vi "configure.vi"(8 "error in (no error)":errorcluster, 11 "ImagingModeDL100901FlexTrajectory in":refnum<class "ImagingModeDL100901FlexTrajectory.lvclass">) -> (0 "error out":errorcluster, 3 "ImagingModeDL100901FlexTrajectory out":refnum<class "ImagingModeDL100901FlexTrajectory.lvclass">)   [LabVIEW 2010, in "ImagingModeDL100901FlexTrajectory.lvclass"]
doc: "The dynamic dispatch version of this VI loads and displays the configuration file associated with the plug-in object. The user modify and save the configuration data."
uses:
  ImagingModeDL100901FlexTrajectory.lvclass
  ImagingModeDL090923Scaffold/ImagingModeDL090923Scaffold/configuration_visibility_cluster.ctl
  ImagingModeDL090923Scaffold/ImagingModeDL090923Scaffold/component_configuration_visibility_cluster.ctl
  ImagingModeDL090923Scaffold/ImagingModeDL090923Scaffold/ImagingModeDL090923Scaffold.lvclass
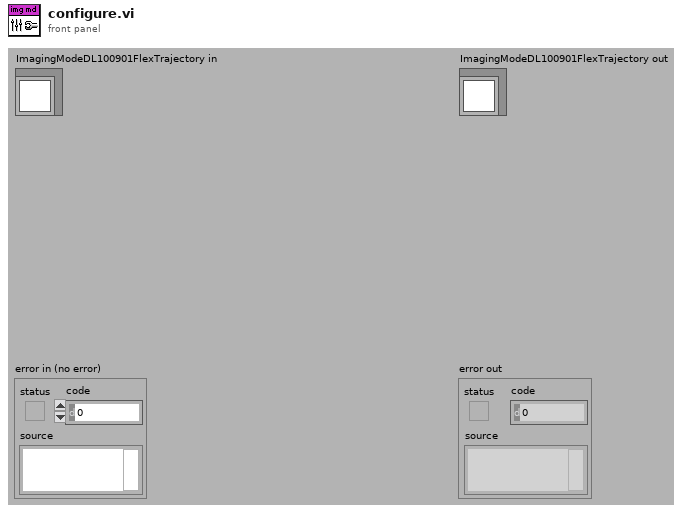
[diagram p1: front panel]
types:
  T1 = typedef "ImagingModeDL090923Scaffold.lvclass/configuration_visibility_cluster.ctl" = cluster{"Instrument":T2, "Trajectory":T2, "ScanHead":T2, "DAQ":T2, "ImageAssembler":T2, "DataCollection":T2, "Display":T2, "Analyser":T2, "Stimulator":T2, "enable Trajectory-to-ImageAssembler adapter":bool}
  T2 = typedef "ImagingModeDL090923Scaffold.lvclass/component_configuration_visibility_cluster.ctl" = cluster{"enable":bool, "enable adapter":bool}
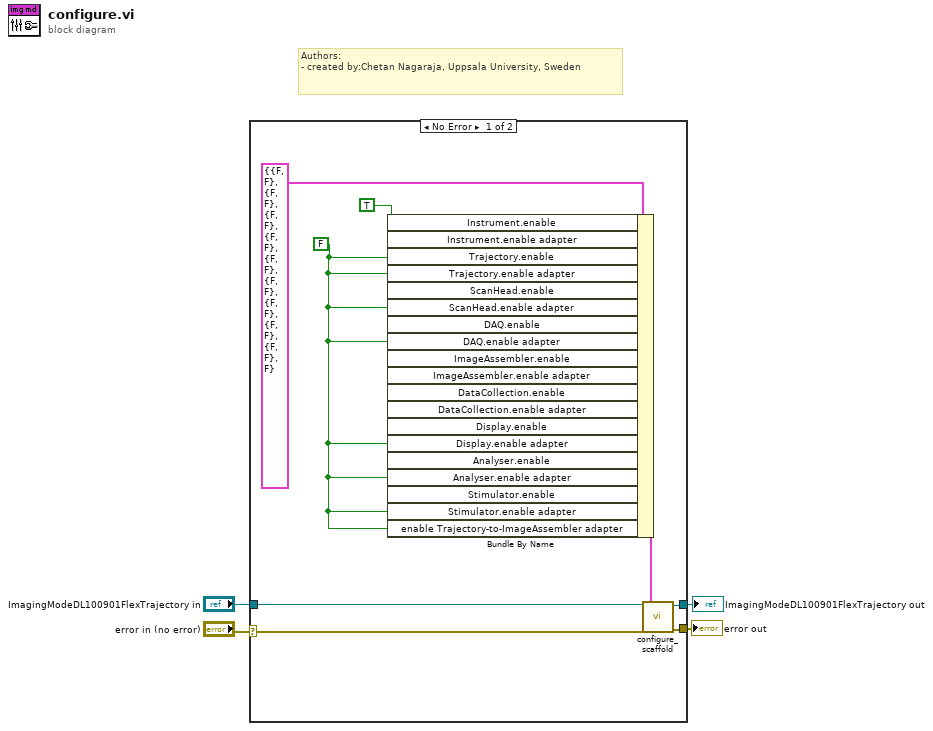
[diagram p0: block diagram]
diagram:
  # "Authors: \n- created by:Chetan Nagaraja, Uppsala University, Sweden"
  n1 = case shown="No Error" "error in (no error)" {
    selector: "error in (no error)" -> [w8 w13]
    tunnel: [w9 w13] -> w4
    tunnel: [w10 w14] -> w3
    tunnel: "ImagingModeDL100901FlexTrajectory in" -> [w11 w14]
    frame No Error {
      w5 = FALSE
      w6 = TRUE
      n2 = Bundle By Name(cluster=T1 {"Instrument"={"enable"=FALSE, "enable adapter"=FALSE}, "Trajectory"={"enable"=FALSE, "enable adapter"=FALSE}, "ScanHead"={"enable"=FALSE, "enable adapter"=FALSE}, "DAQ"={"enable"=FALSE, "enable adapter"=FALSE}, "ImageAssembler"={"enable"=FALSE, "enable adapter"=FALSE}, "DataCollection"={"enable"=FALSE, "enable adapter"=FALSE}, "Display"={"enable"=FALSE, "enable adapter"=FALSE}, "Analyser"={"enable"=FALSE, "enable adapter"=FALSE}, "Stimulator"={"enable"=FALSE, "enable adapter"=FALSE}, "enable Trajectory-to-ImageAssembler adapter"=FALSE} ("visibilities"), "Instrument.enable"=w6, "Instrument.enable adapter"=w5, "Trajectory.enable"=w6, "Trajectory.enable adapter"=w5, "ScanHead.enable"=w6, "ScanHead.enable adapter"=w5, "DAQ.enable"=w6, "DAQ.enable adapter"=w5, "ImageAssembler.enable"=w6, "ImageAssembler.enable adapter"=w6, "DataCollection.enable"=w6, "DataCollection.enable adapter"=w6, "Display.enable"=w6, "Display.enable adapter"=w5, "Analyser.enable"=w6, "Analyser.enable adapter"=w5, "Stimulator.enable"=w6, "Stimulator.enable adapter"=w5, "enable Trajectory-to-ImageAssembler adapter"=w5) -> (w7:T1)
      n3 = call-dynamic "configure_scaffold.vi"("error in (no error)"=w8, "visibilities"=w7, "ScanModeDL090923Scaffold in"=w11) -> ("error out"=w9:errorcluster, "ScanModeDL090923Scaffold out"=w10:refnum<class "ImagingModeDL100901FlexTrajectory.lvclass">)  [unwired: 7 in]
    }
    frame Error {
    }
  }
  "error out" <- w4
  "ImagingModeDL100901FlexTrajectory out" <- w3
